vi "Pracownia7.vi"() -> ()   [LabVIEW 2019]
uses:
  <vilib>/Platform/TimedLoop/XDataNode/timing_clust.ctl
  <vilib>/Platform/TimedLoop/XDataNode/nitl_modes.ctl
  <vilib>/Platform/TimedLoop/XDataNode/wakeup.ctl
  <vilib>/Platform/TimedLoop/scheduler/LVUserAPI/_suppVIs/Create_1kHz_TSource.vi
  <vilib>/Platform/TimedLoop/XDataNode/XDataNode.xnode
  <vilib>/Platform/TimedLoop/XDataNode/XDNodeRunTimeDep.lvlib
panel:
  in  "Synchronizacja":bool
  out "?":bool
  out "L2 Stop":dbl
  out "L2 End":i64
  out "Iteracja pêtli 2":i32
  out "Error 2":errorcluster
  out "L1 Stop":dbl
  out "czas_pocz":dbl
  out "?":bool
  out "Iteracja pêtli 1":i32
  out "L1 End":i64
  in  "Okres pêtli [s]":dbl=0.5 min=0.5 max=20.0 step=0.5
  out "S0 End":i64
  out "S0 Start":i64
  out "Error 1":errorcluster
  # "K\nO\nN\nI\nE\nC"
  # "NIE"
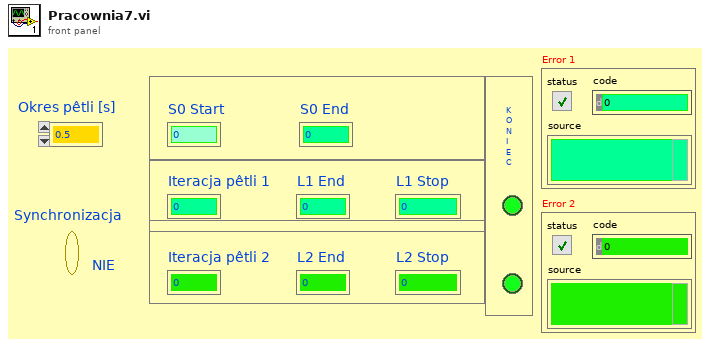
[diagram p1: front panel]
types:
  T1 = typedef "XDNodeRunTimeDep.lvlib/timing_clust.ctl" = cluster{"Expected End [f-1]":u64, "Actual End [f-1]":u64, "Finished Late? [f-1]":bool, "Expected End [i-1]":u64, "Actual End [i-1]":u64, "Finished Late? [i-1]":bool, "Expected Start [i]":u64, "Actual Start [i]":u64, "Expected Start [f]":u64, "Actual Start [f]":u64, "Source Name":string, "Structure Name":string, "Period":i64, "Deadline":i64, "Offset":i64, "Start":i64, "Priority":i32, "Timeout":i32, "Mode":T2, "Wakeup Reason":T3, "Error":errorcluster, "Source Type":string, "Secondary Source Type":string, "Global End Time":u64, "Global Start Time":u64, "Frame Duration":u64, "Iteration Duration":u64, "Assigned CPU":i32, "I/O Scan Engine Mode":u32}
  T2 = typedef "XDNodeRunTimeDep.lvlib/nitl_modes.ctl" = enum32{"No Change", "Process missed periods, maintain original phase", "Discard missed periods, maintain original phase", "Process missed periods, ignore original phase", "Discard missed periods, ignore original phase"}
  T3 = typedef "XDNodeRunTimeDep.lvlib/wakeup.ctl" = enum32{"Normal", "Aborted", "Asynchronous wakeup", "Timing source error", "Timed loop error", "Timeout"}
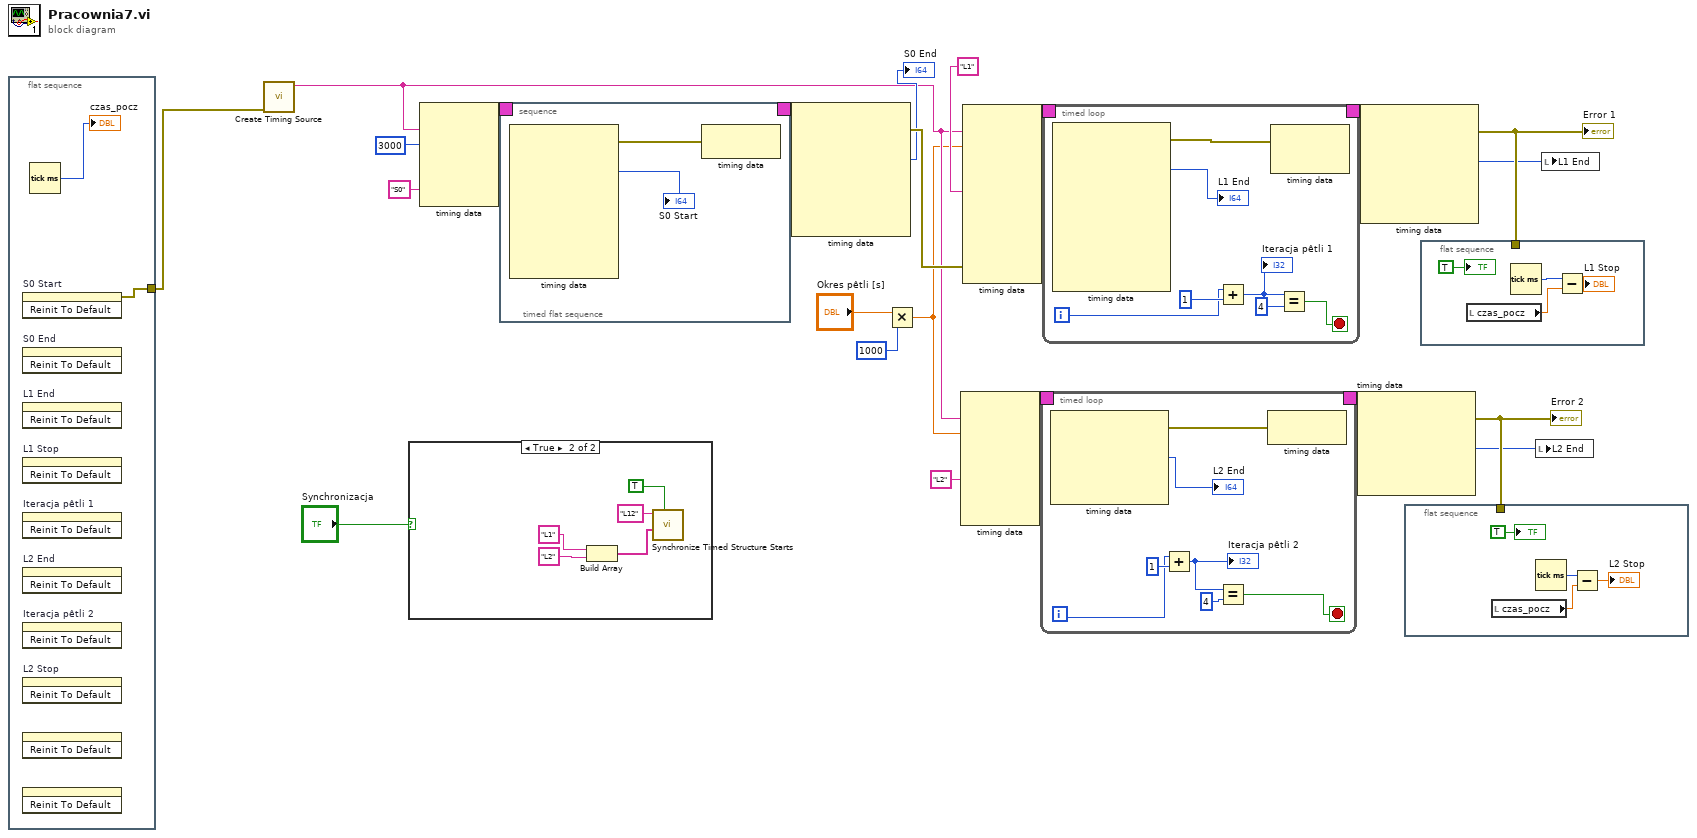
[diagram p0: block diagram]
diagram:
  n1 = flat-sequence {
    tunnel: [w23] -> w3
    frame #0 {
      n2 = invoke on="S0 Start" class="DigNum (strict)" method="Reinit To Default"() -> (error out=w23:errorcluster)  [unwired: 3 in, 2 out]
      n3 = invoke on="S0 End" class="DigNum (strict)" method="Reinit To Default"() -> ()  [unwired: 3 in, 3 out]
      n4 = invoke on="L1 End" class="DigNum (strict)" method="Reinit To Default"() -> ()  [unwired: 3 in, 3 out]
      n5 = invoke on="L1 Stop" class="DigNum (strict)" method="Reinit To Default"() -> ()  [unwired: 3 in, 3 out]
      n6 = invoke on="Iteracja pêtli 1" class="DigNum (strict)" method="Reinit To Default"() -> ()  [unwired: 3 in, 3 out]
      n7 = invoke on="L2 End" class="DigNum (strict)" method="Reinit To Default"() -> ()  [unwired: 3 in, 3 out]
      n8 = invoke on="Iteracja pêtli 2" class="DigNum (strict)" method="Reinit To Default"() -> ()  [unwired: 3 in, 3 out]
      n9 = invoke on="L2 Stop" class="DigNum (strict)" method="Reinit To Default"() -> ()  [unwired: 3 in, 3 out]
      n10 = invoke class="Bool (strict)" method="Reinit To Default"() -> ()  [unwired: 3 in, 3 out]
      n11 = invoke class="Bool (strict)" method="Reinit To Default"() -> ()  [unwired: 3 in, 3 out]
      n12 = Tick Count (ms)() -> (millisecond timer value=→"czas_pocz":u32)
    }
  }
  n13 = call-poly <vilib>:"Create Timing Source.vi"("error in (no error)"=w3) -> ("name (out)"=w6:string)  [unwired: 9 in, 1 out]
  n14 = case shown="True" "Synchronizacja" {
    frame False {
    }
    frame True {
      n15 = Build Array("L1", "L2") -> (w25:string[])
      n16 = call <vilib>:"Synchronize Timed Structure Starts.vi"("replace (T)"=TRUE, "timed structure names"=w25, "synchronization group name"="L12") -> ()  [unwired: 7 in, 2 out]
    }
  }
  n17 = node-c288(w6, i64 3000 ("Offset"), "S0" ("Structure Name")) -> (w22:T1)  [unwired: 2 in]
  n18 = timed-sequence {
    timing: w22 -> [_]
    timing-out: [_] -> w21
    n19 = timed-flat-sequence {
      n20 = node-c288() -> (w31:errorcluster, →"S0 Start":i64)  [unwired: 1 in, 7 out]
      n21 = node-c288(w31) -> ()  [unwired: 1 out]
    }
  }
  n22 = node-c288(w21) -> (w18:errorcluster, →"S0 End":i64)  [unwired: 5 out]
  n23 = Multiply(x="Okres pêtli [s]", y=i64 1000) -> (x*y=w5:dbl)
  n24 = node-c288(w6, w5, "L2" ("Structure Name")) -> (w9:T1)  [unwired: 4 in]
  n25 = node-c288(w6, w5, "L1" ("Structure Name"), w18) -> (w20:T1)  [unwired: 6 in]
  n26 = timed-loop {
    timing: w9 -> [_]
    timing-out: [_] -> w8
    i -> [w40]
    stop <- w41 stop-if-true
    n27 = node-c288() -> (w44:errorcluster, →"L2 End":i64)  [unwired: 1 in, 3 out]
    n28 = Add(x=w40, y=1) -> (x+y=w39:i32)
    "Iteracja pêtli 2" <- w39
    n29 = Equal?(x=w39, y=4) -> (x = y?=w41:bool)
    n30 = node-c288(w44) -> ()  [unwired: 1 out]
  }
  n31 = timed-loop {
    timing: w20 -> [_]
    timing-out: [_] -> w19
    i -> [w54]
    stop <- w51 stop-if-true
    n32 = node-c288() -> (w57:errorcluster, →"L1 End":i64)  [unwired: 1 in, 8 out]
    n33 = Add(x=w54, y=1) -> (x+y=w53:i32)
    "Iteracja pêtli 1" <- w53
    n34 = node-c288(w57) -> ()  [unwired: 1 in, 1 out]
    n35 = Equal?(x=w53, y=4) -> (x = y?=w51:bool)
  }
  n36 = node-c288(w8) -> (w4:errorcluster, w1:i64)  [unwired: 3 out]
  "Error 2" <- w4
  n37 = node-c288(w19) -> (w17:errorcluster, w10:i64)  [unwired: 4 out]
  "Error 1" <- w17
  n38 = flat-sequence {
    tunnel: w4 -> [_]
    frame #0 {
      n39 = local read "czas_pocz"() -> (w66:dbl)
      n40 = Tick Count (ms)() -> (millisecond timer value=w67:u32)
      n41 = Subtract(x=w67, y=w66) -> (x-y=→"L2 Stop":dbl)
      "?" <- TRUE
    }
  }
  n42 = flat-sequence {
    tunnel: w17 -> [_]
    frame #0 {
      n43 = local read "czas_pocz"() -> (w69:dbl)
      n44 = Tick Count (ms)() -> (millisecond timer value=w70:u32)
      n45 = Subtract(x=w70, y=w69) -> (x-y=→"L1 Stop":dbl)
      "?" <- TRUE
    }
  }
  n46 = local write "L2 End"(w1) -> ()
  n47 = local write "L1 End"(w10) -> ()
